vi "Map2.vi"(8 "地图比例":u8(slide)=3 min=3 max=18 step=1 scale=6.0..18.0, 10 "纬度":string, 11 "经度":string) -> (2 "BaiduMapURL":string)   [LabVIEW 2018]
panel:
  out "最新经纬度":string
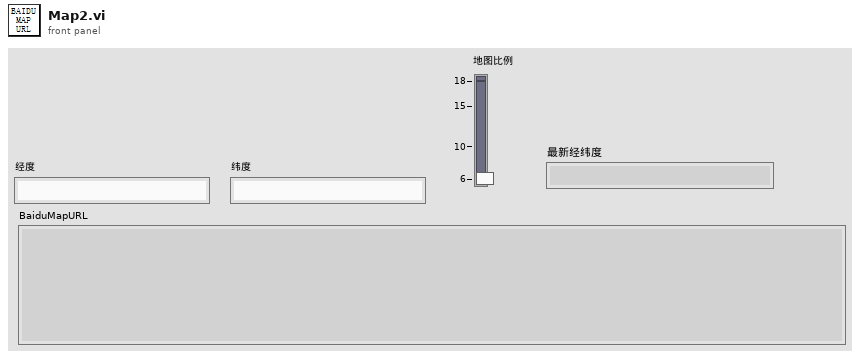
[diagram p1: front panel]
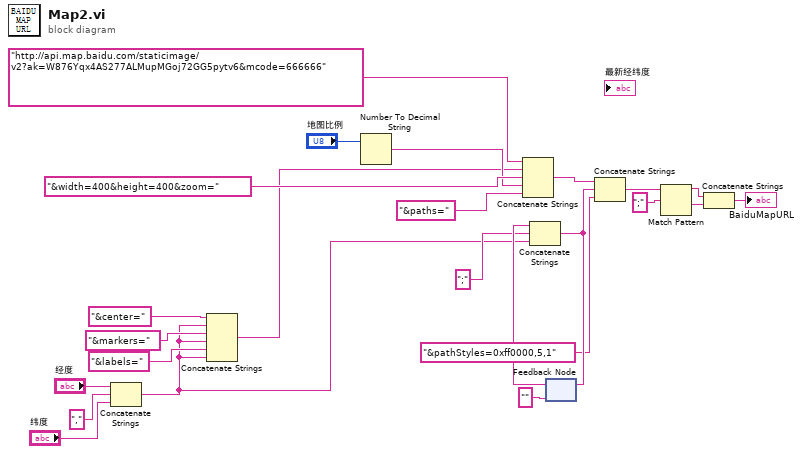
[diagram p0: block diagram]
diagram:
  n1 = Concatenate Strings("经度", ",", "纬度") -> (w1:string)
  n2 = Concatenate Strings("&center=", w1, "&markers=", w1, "&labels=", w1) -> (w2:string)
  n3 = Number To Decimal String(number="地图比例") -> (decimal integer string=w18:string)  [unwired: 1 in]
  n4 = Concatenate Strings("http://api.map.baidu.com/staticimage/v2?ak=W876Yqx4AS277ALMupMGoj72GG5pytv6&mcode=666666", w2, "&width=400&height=400&zoom=" ("字符串"), w18, "&paths=") -> (w15:string)
  n5 = feedback #1("") -> (w17:string)
  n6 = Concatenate Strings(w17, ";" ("字符串"), w1) -> (w14:string)
  n7 = feedback-in #1(w14) -> ()
  n8 = Concatenate Strings(w15, w14, "&pathStyles=0xff0000,5,1" ("字符串")) -> (w9:string)
  n9 = Match Pattern(string=w9, regular expression=";" ("正则表达式")) -> (before substring=w11:string, after substring=w10:string)  [unwired: 1 in, 2 out]
  n10 = Concatenate Strings(w11, w10) -> (→"BaiduMapURL":string)
